vi "SetSettings_NoFile_CreatesFile.vi"(9 "Expected":string="Test.lvlib", 10 "Value":string="ProjectLibrarySuffix", 11 "Name":string="ProjectLibrarySuffix") -> (0 "error out":errorcluster)   [LabVIEW 2017, in "Configuration.Tests.lvlib"]
uses:
  Configuration.Tests.lvlib
  0a18371b-3929-4a79-b65e-3270324a61a8.vi
  Constraint/IsEqual/Create.vi
  Constraint/IsEqual/IsEqual.lvclass
  Configuration/Configuration.lvlib
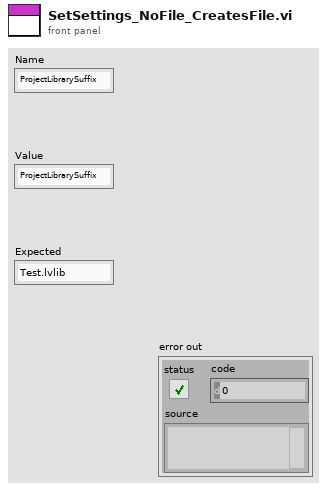
[diagram p1: front panel]
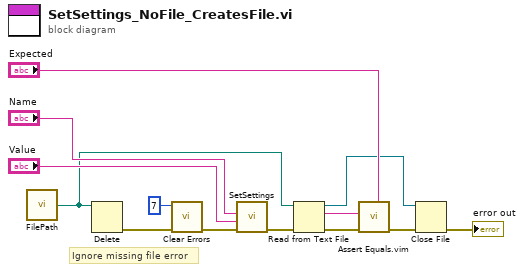
[diagram p0: block diagram]
diagram:
  # "Ignore missing file error"
  n1 = call "FilePath.vi"() -> ("File Path"=w4:path)
  n2 = Delete(path (use dialog)=w4) -> (error out=w3:errorcluster)  [unwired: 4 in, 2 out]
  n3 = call <vilib>:"Clear Errors.vi"("error in (no error)"=w3, "specific error code to clear (0: all)"=7) -> ("error out"=w2:errorcluster)  [unwired: 4 in, 1 out]
  n4 = call "SetSettings.vi"("error in (no error)"=w2, "Value"="Value", "Name"="Name") -> ("error out"=w13:errorcluster)  [unwired: 8 in]
  n5 = Read from Text File(file (use dialog)=w4, error in=w13) -> (refnum out=w7:refnum<file>, text=w5:string, error out=w9:errorcluster)  [unwired: 2 in, 1 out]
  n6 = call "Assert Equals.vim"("Expected"="Expected", "error in (no error)"=w9, "Actual"=w5) -> ("error out"=w11:errorcluster)  [unwired: 8 in]
  n7 = Close File(refnum=w7, error in=w11) -> (error out=→"error out":errorcluster)  [unwired: 1 out]
